vi "Get Triggered Block.vi"(8 "error in (no error)":errorcluster, 9 "Post-trigger points":i32, 10 "Pre-trigger points":i32, 11 "RP Instrument in":refnum<class "RP Instrument.lvclass">) -> (0 "error out":errorcluster, 2 "Data out":string, 3 "RP Instrument out":refnum<class "RP Instrument.lvclass">)   [LabVIEW 2019, in "RP Instrument.lvclass"]
uses:
  RP Instrument.lvclass
  RP Instrument.lvclass/RP Instrument.ctl
  RP Communicator/RP Communicator.lvclass
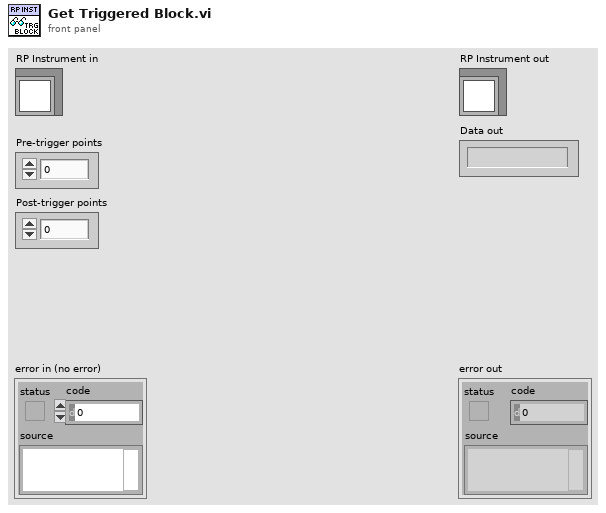
[diagram p1: front panel]
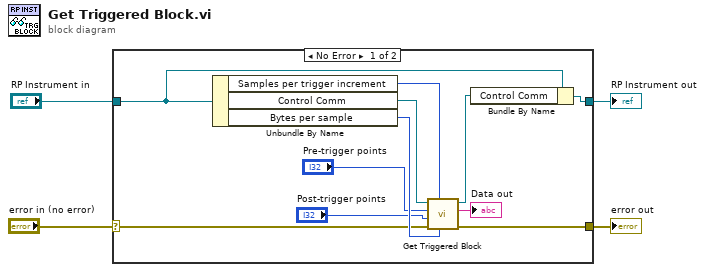
[diagram p0: block diagram]
diagram:
  n1 = case shown="No Error" "error in (no error)" {
    selector: "error in (no error)" -> [w9 w17]
    tunnel: [w8 w17] -> w3
    tunnel: [w11 w16] -> w1
    tunnel: "RP Instrument in" -> [w12 w16]
    frame No Error {
      n2 = Unbundle By Name(w12) -> ("Samples per trigger increment"=w5:i32, "Control Comm"=w15:refnum<class "RP Communicator.lvclass">, "Bytes per sample"=w13:i32)
      n3 = call-dynamic "Get Triggered Block.vi"("Bytes per sample"=w13, "Samples per trigger increment"=w5, "error in (no error)"=w9, "Post-trigger samples"="Post-trigger points", "Pre-trigger samples"="Pre-trigger points", "RP Communicator in"=w15) -> ("error out"=w8:errorcluster, "data out"=→"Data out":string, "RP Communicator out"=w14:refnum<class "RP Communicator.lvclass">)  [unwired: 3 in]
      n4 = Bundle By Name(cluster=w12, "Control Comm"=w14) -> (w11:refnum<class "RP Instrument.lvclass">)
    }
    frame Error {
    }
  }
  "error out" <- w3
  "RP Instrument out" <- w1
